vi "Group Type.vi"(8 "error in (no error)":errorcluster, 11 "Group in":refnum<class "Group Config.lvclass">) -> (0 "error out":errorcluster, 2 "Group Data Type":T1, 3 "Group out":refnum<class "Group Config.lvclass">)   [LabVIEW 2020, in "VolatusConfig.lvlib" / "Group Config.lvclass"]
uses:
  Group Config.lvclass
  C:/dev/lv20CE/relink/lv-volatus/VolatusConfig/VolatusConfigElement/VolatusConfigElement.lvclass
  Meta Name.ctl
  VolatusConfigElement/VolatusConfigElement.lvclass/VolatusConfigElement.ctl
  Group Config.lvclass/Group Config.ctl
  lv-cdm/CDM-Config/Config Element/Config Element.lvclass
  VolatusConfig.lvlib
  VolatusConfigElement/VolatusConfigElement.lvclass
  lv-vecto/Vecto/Group Data Type.ctl
  lv-vecto/VectoConfig/VectoConfig.lvlib
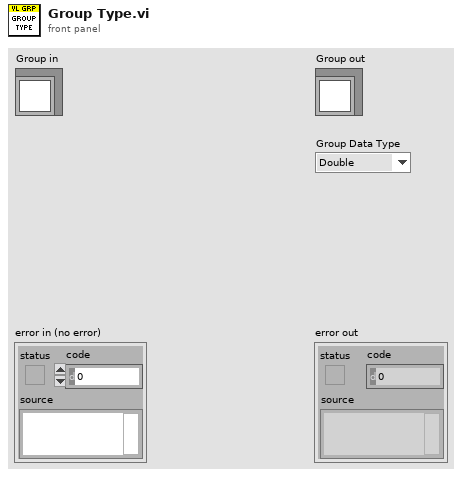
[diagram p1: front panel]
types:
  T1 = typedef "VectoConfig.lvlib/Group Data Type.ctl" = enum16{"Double", "String", "Bool"}
  T2 = typedef "VolatusConfig.lvlib/Meta Name.ctl" = enum16{"VL_Type", "VL_Node_IP", "VL_Node_Type", "VL_Task_Type", "VL_Group_Type", "VL_Channel_Type", "VL_Channel_DataType", "VL_Config_Version", "VL_Overlay_Type", "VL_Config_Hash"}
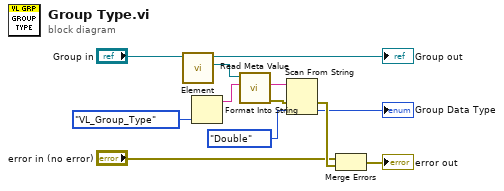
[diagram p0: block diagram]
diagram:
  n1 = call "Element.vi"("VolatusConfigElement in"="Group in") -> ("Element"=w1:refnum<class "Config Element.lvclass">, "VolatusConfigElement out"=→"Group out":refnum<class "Group Config.lvclass">)  [unwired: 9 in]
  n2 = Format Into String(Meta_Name."VL_Group_Type" ("Meta Name")) -> (resulting string=w4:string)  [unwired: 3 in, 1 out]
  n3 = call "Read Meta Value.vi"("Meta Name"=w4, "Config Element in"=w1) -> ("error out"=w6:errorcluster, "Meta Value"=w9:string)  [unwired: 7 in, 1 out]
  n4 = Scan From String(input string=w9, error in=w6, default 1=Group_Data_Type."Double" ("Group Data Type")) -> (error out=w12:errorcluster, output 1=→"Group Data Type":T1)  [unwired: 2 in, 2 out]
  n5 = Merge Errors("error in (no error)", w12) -> (→"error out":errorcluster)
